vi "IsBaseClass.vi"(0 "RefIn":refnum<class "ClassWriterNative.lvclass">, 1 "LvClass":refnum<vi>, 5 "error in":errorcluster) -> (14 "RefOut":refnum<class "ClassWriterNative.lvclass">, 15 "BaseClass":bool, 19 "error out":errorcluster)   [LabVIEW 2014, in "ClassWriterNative.lvclass"]
uses:
  <resource>/Framework/Providers/Open_GDS/ClassProviders/Provider_LvNativeClass/ClassWriterNative_class/ClassWriterNative.lvclass
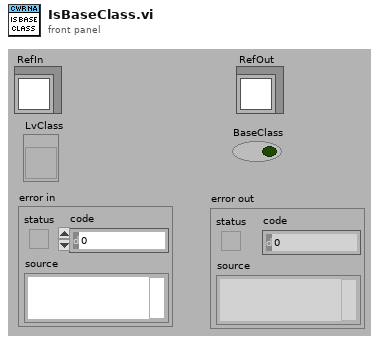
[diagram p1: front panel]
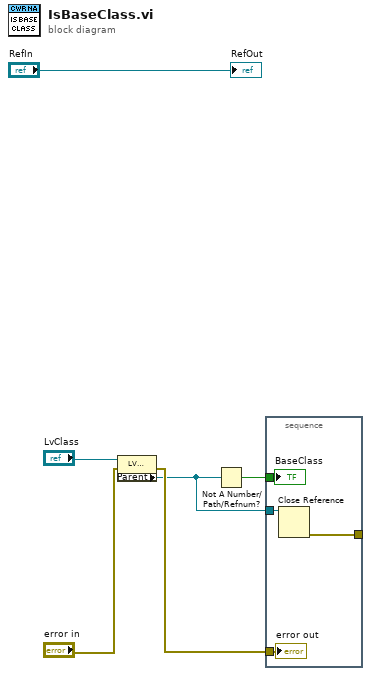
[diagram p0: block diagram]
diagram:
  n1 = property class="LVClassLibrary"(reference="LvClass", error in="error in") -> (error out=w2:errorcluster, "Parent"=w1:refnum<vi>)  [unwired: 1 out]
  n2 = Not A Number/Path/Refnum?(number/path/refnum=w1) -> (NaN/Path/Refnum?=w6:bool)
  n3 = stacked-sequence {
    tunnel: w6 -> [w10]
    tunnel: w2 -> [w9]
    tunnel: w1 -> [w8]
    tunnel: [w7] -> _
    frame #0 {
      n4 = Close Reference(reference=w8) -> (error out=w7:errorcluster)  [unwired: 1 in]
      "BaseClass" <- w10
      "error out" <- w9
    }
  }
  "RefOut" <- "RefIn"
